vi "Run.vi"(8 "error in (no error)":errorcluster, 11 "Runnable In":refnum<class "Runnable.lvclass">) -> (0 "error out":errorcluster, 1 "Done?":bool, 2 "Results":T1[](array[typedef]), 3 "Runnable Out":refnum<class "Runnable.lvclass">)   [LabVIEW 2020, in "Runnable.lvclass"]
uses:
  Runnable.lvclass
  Result/Result.ctl
  Result/Status.ctl
  Result/Type.ctl
  Result/Result.lvlib
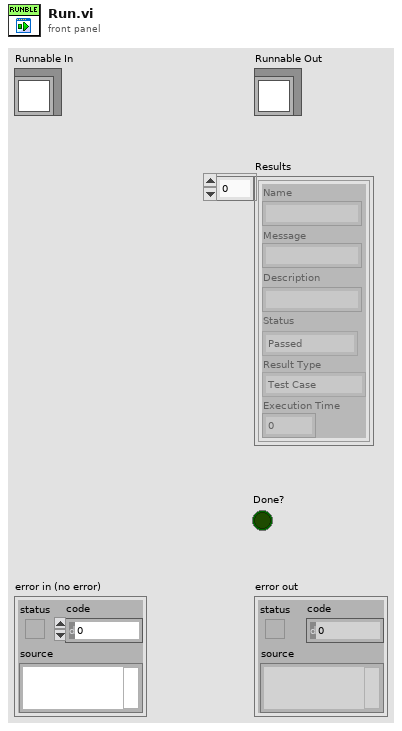
[diagram p1: front panel]
types:
  T1 = typedef "Result.lvlib/Result.ctl" = cluster{"Name":string, "Message":string, "Description":string, "Status":T2, "Result Type":T3, "Execution Time":dbl}
  T2 = typedef "Result.lvlib/Status.ctl" = enum16{"", "Passed", "Failed", "Error", "Skipped", "Setup Error", "Broken", "Teardown Error"}
  T3 = typedef "Result.lvlib/Type.ctl" = enum16{"Test Case", "Test Suite", "Test Run", "Pass", "Fail", "Skip", "Pass if", "Fail if", "Pass if Error", "Fail if Error", "Pass if Equal", "Fail if Equal"}
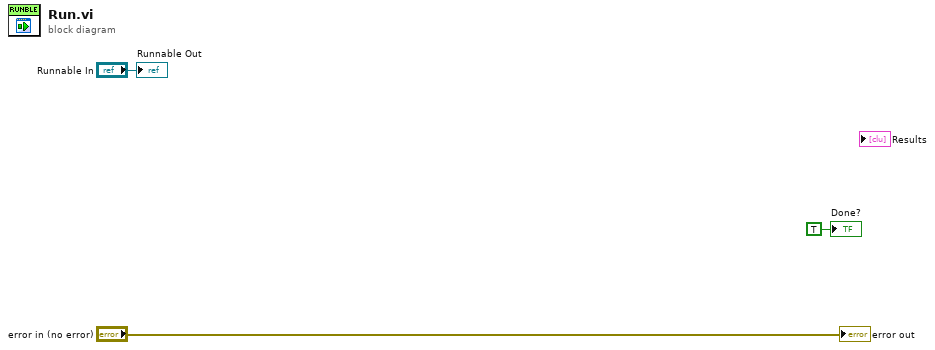
[diagram p0: block diagram]
diagram:
  "error out" <- "error in (no error)"
  "Done?" <- TRUE ("Done?")
  "Runnable Out" <- "Runnable In"
